vi "Get Tree Indentation Levels Recursive.vi"(8 "error in (no error)":errorcluster, 10 "Initial tree level":i32, 11 "Message Array":refnum<class "Message.lvclass">[](array[class])) -> (0 "error out":errorcluster, 2 "Tree indentation level Array":i32[](array[numeric]), 3 "Class Base Name Array":string[](array[string]))   [LabVIEW 2020, in "Sequencer.lvlib"]
doc: "Recursivly get Class Base Names and indentation levels through nested Batch Msg's."
uses:
  Sequencer.lvlib
  PPL/HDH.Actor Framework.Core.Actor.lvlibp/1abvi3w/vi.lib/ActorFramework/Message/Message.lvclass
  Sequencer Messages/Batch Msg/Batch Msg.lvclass
  Sequencer Messages/Batch Msg/Batch Msg.lvclass/Batch Msg.ctl
  PPL/HDH.Data.Generic.lvlibp
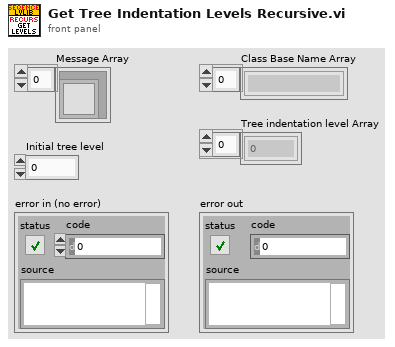
[diagram p1: front panel]
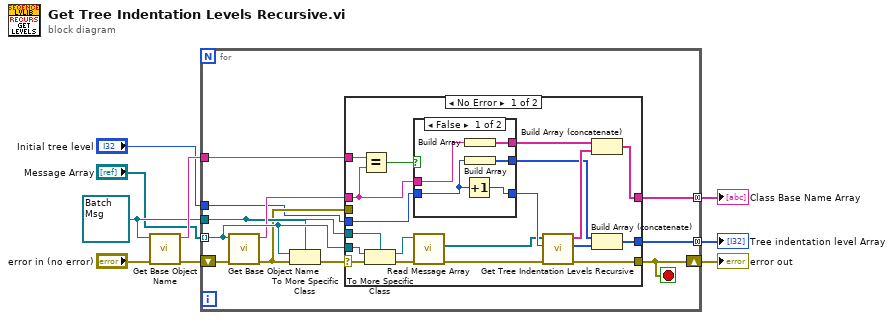
[diagram p0: block diagram]
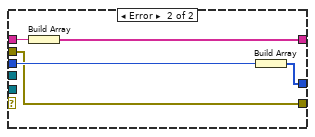
[diagram p3: hidden frame]
diagram:
  w3 = refnum<class "Batch Msg.lvclass"> refnum ("Sequencer.lvlib:Batch Msg.lvclass")
  n1 = call "Get Base Object Name.vi"("error in (no error)"="error in (no error)", "Object in"=w3) -> ("error out"=w5:errorcluster, "Base class name"=w4:string)  [unwired: 8 in]
  n2 = for {
    tunnel: "Message Array" -> [w17] mode=indexing
    tunnel: w3 -> [w14]
    tunnel: [w19] -> w8 mode=concatenating
    tunnel: [w18] -> w9 mode=concatenating
    tunnel: w4 -> [w15]
    shift-right: [w11] -> w7
    shift-left: w5 -> [w13]
    tunnel: "Initial tree level" -> [w10]
    stop <- w11 stop-if-true
    n3 = call "Get Base Object Name.vi"("error in (no error)"=w13, "Object in"=w17) -> ("error out"=w12:errorcluster, "Base class name"=w16:string)  [unwired: 8 in]
    n4 = To More Specific Class(target class=w14, reference=w17, error in=w12) -> (error out=w20:errorcluster)  [unwired: 1 out]
    n5 = case shown="No Error" w20 {
      selector: w20 -> [w35 _]
      tunnel: w10 -> [w32 w50]
      tunnel: w17 -> [w37 _]
      tunnel: [w26 w49] -> w19
      tunnel: [w21 w48] -> w18
      tunnel: w16 -> [w29 w47]
      tunnel: w15 -> [w39 _]
      tunnel: w14 -> [w36 _]
      tunnel: [w24 w46] -> w11
      tunnel: w12 -> [_ w46]
      frame No Error {
        n6 = Equal?(x=w39, y=w29) -> (x = y?=w38:bool)
        n7 = To More Specific Class(target class=w36, reference=w37, error in=w35) -> (specific class reference=w34:refnum<class "Batch Msg.lvclass">, error out=w33:errorcluster)
        n8 = case shown="False" w38 {
          tunnel: [w44 w45] -> w31
          tunnel: w32 -> [w42 w45]
          tunnel: w29 -> [w43 _]
          tunnel: [w41 _] -> w28
          tunnel: [w40 _] -> w23
          frame False {
            n9 = Increment(x=w42) -> (x+1=w44:i32)
            n10 = Build Array(w43) -> (w41:string[])
            n11 = Build Array(w42) -> (w40:i32[])
          }
          frame True {
          }
        }
        n12 = call "Read Message Array.vi"("error in (no error)"=w33, "Batch Msg in"=w34) -> ("error out"=w25:errorcluster, "Message Array"=w30:refnum<class "Message.lvclass">[])  [unwired: 7 in, 1 out]
        n13 = call "Get Tree Indentation Levels Recursive.vi"("error in (no error)"=w25, "Initial tree level"=w31, "Message Array"=w30) -> ("error out"=w24:errorcluster, "Tree indentation level Array"=w22:i32[], "Class Base Name Array"=w27:string[])  [unwired: 6 in]
        n14 = Build Array (concatenate)(w28, w27) -> (w26:string[])
        n15 = Build Array (concatenate)(w23, w22) -> (w21:i32[])
      }
      frame Error {
        n16 = Build Array(w47) -> (w49:string[])
        n17 = Build Array(w50) -> (w48:i32[])
      }
    }
  }
  "Tree indentation level Array" <- w9
  "Class Base Name Array" <- w8
  "error out" <- w7
